vi "GUI.Stream.Disable.vi"(8 "error in (no error)":errorcluster, 11 "State Variables in":T1) -> (0 "error out":errorcluster)   [LabVIEW 2025, in "XNET Bus Monitor Client.lvlib"]
uses:
  XNET Bus Monitor Client.lvlib
  <vilib>/Utility/miscctls.llb/LVRowAndColumnUnsignedTypeDef.ctl
  Types/GUI.StateVariables.ctl
  Types/StreamEngine.CmdQueueData.ctl
  Types/StreamEngine.CmdQueueData.Cmd.ctl
  Types/StreamEngine.QueueRefs.ctl
  Types/GUI.Controls.Refs.ctl
  <vilib>/gRPC/LabVIEW gRPC Library/Shared/grpcId.ctl
  <vilib>/gRPC/LabVIEW gRPC Library/grpc-lvsupport-release.lvlib
  xnet_can_bus_monitor_api_client/RPC Messages/ni_xnet_can_bm_api_DirectionFilter.ctl
  xnet_can_bus_monitor_api_client/xnet_can_bus_monitor_api_client.lvlib
  xnet_can_bus_monitor_api_client/RPC Messages/ni_xnet_can_bm_api_FrameFilter.ctl
  Types/gRPC.ConnectionInfo.ctl
  Types/SubProcessEngine.CmdQueueData.ctl
  Types/SubProcessEngine.CmdQueueData.Cmd.ctl
  Types/SubProcessEngine.QueueRefs.ctl
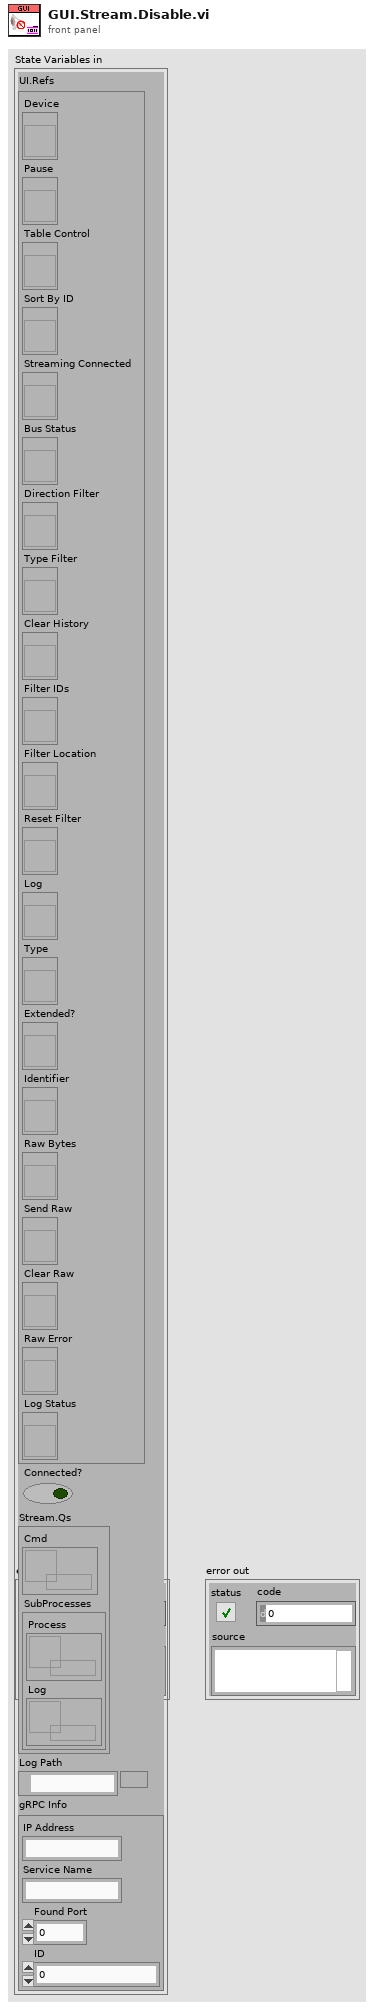
[diagram p1: front panel]
types:
  T1 = typedef "XNET Bus Monitor Client.lvlib/GUI.StateVariables.ctl" = cluster{"UI.Refs":T2, "Connected?":bool, "Stream.Qs":T3, "Log Path":path, "gRPC Info":T5}
  T2 = typedef "XNET Bus Monitor Client.lvlib/GUI.Controls.Refs.ctl" = cluster{"Device":refnum<vi>, "Pause":refnum<vi>, "Table Control":refnum<vi>, "Sort By ID":refnum<vi>, "Streaming Connected":refnum<vi>, "Bus Status":refnum<vi>, "Direction Filter":refnum<vi>, "Type Filter":refnum<vi>, "Clear History":refnum<vi>, "Filter IDs":refnum<vi>, "Filter Location":refnum<vi>, "Reset Filter":refnum<vi>, "Log":refnum<vi>, "Type":refnum<vi>, "Extended?":refnum<vi>, "Identifier":refnum<vi>, "Raw Bytes":refnum<vi>, "Send Raw":refnum<vi>, "Clear Raw":refnum<vi>, "Raw Error":refnum<vi>, "Log Status":refnum<vi>}
  T3 = typedef "XNET Bus Monitor Client.lvlib/StreamEngine.QueueRefs.ctl" = cluster{"Cmd":refnum<queue>, "SubProcesses":T4}
  T4 = typedef "XNET Bus Monitor Client.lvlib/SubProcessEngine.QueueRefs.ctl" = cluster{"Process":refnum<queue>, "Log":refnum<queue>}
  T5 = typedef "XNET Bus Monitor Client.lvlib/gRPC.ConnectionInfo.ctl" = cluster{"IP Address":string, "Service Name":string, "Found Port":u64, "ID":T6}
  T6 = typedef "grpc-lvsupport-release.lvlib/grpcId.ctl" = u64
  T7 = enum16{"CAN Data", "CAN Remote", "CAN Bus Error", "CAN 2.0 Data", "CAN FD Data", "CAN FD+BRS Data", "J1939 Data", "Delay", "Log Trigger", "Start Trigger"}
  T8 = typedef "LVRowAndColumnUnsignedTypeDef.ctl" = cluster{"Row":u32, "Column":u32}
  T9 = enum8{"Enabled", "Disabled", "Disabled and Grayed Out"}
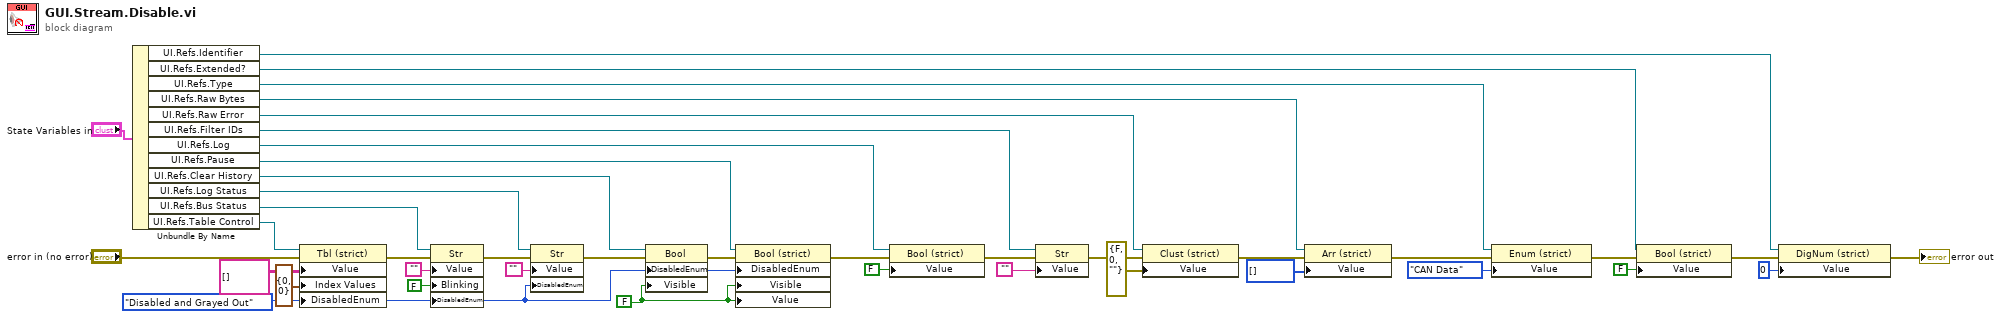
[diagram p0: block diagram]
diagram:
  w30 = FALSE ("Value")
  w3 = T9."Disabled and Grayed Out" ("Disabled")
  n1 = Unbundle By Name("State Variables in") -> ("UI.Refs.Identifier"=w14:refnum<vi>, "UI.Refs.Extended?"=w16:refnum<vi>, "UI.Refs.Type"=w18:refnum<vi>, "UI.Refs.Raw Bytes"=w21:refnum<vi>, "UI.Refs.Raw Error"=w22:refnum<vi>, "UI.Refs.Filter IDs"=w24:refnum<vi>, "UI.Refs.Log"=w28:refnum<vi>, "UI.Refs.Pause"=w31:refnum<vi>, "UI.Refs.Clear History"=w33:refnum<vi>, "UI.Refs.Log Status"=w4:refnum<vi>, "UI.Refs.Bus Status"=w37:refnum<vi>, "UI.Refs.Table Control"=w39:refnum<vi>)
  n2 = property class="Tbl (strict)"(reference=w39, error in="error in (no error)", "Value"=string[][] [], "Index Values"=T8 {"Row"=0, "Column"=0}, "DisabledEnum"=w3) -> (error out=w5:errorcluster)  [unwired: 1 out]
  n3 = property class="Str"(reference=w37, error in=w5, "Value"="", "Blinking"=FALSE, "DisabledEnum"=w3) -> (error out=w2:errorcluster)  [unwired: 1 out]
  n4 = property class="Str"(reference=w4, error in=w2, "Value"="", "DisabledEnum"=w3) -> (error out=w1:errorcluster)  [unwired: 1 out]
  n5 = property class="Bool"(reference=w33, error in=w1, "DisabledEnum"=w3, "Visible"=w30) -> (error out=w32:errorcluster)  [unwired: 1 out]
  n6 = property class="Bool (strict)"(reference=w31, error in=w32, "DisabledEnum"=w3, "Visible"=w30, "Value"=w30) -> (error out=w26:errorcluster)  [unwired: 1 out]
  n7 = property class="Bool (strict)"(reference=w28, error in=w26, "Value"=FALSE ("Visible")) -> (error out=w25:errorcluster)  [unwired: 1 out]
  n8 = property class="Str"(reference=w24, error in=w25, "Value"="") -> (error out=w20:errorcluster)  [unwired: 1 out]
  n9 = property class="Clust (strict)"(reference=w22, error in=w20, "Value"=errorcluster {"status"=FALSE, "code"=0, "source"=""}) -> (error out=w19:errorcluster)  [unwired: 1 out]
  n10 = property class="Arr (strict)"(reference=w21, error in=w19, "Value"=u8[] []) -> (error out=w17:errorcluster)  [unwired: 1 out]
  n11 = property class="Enum (strict)"(reference=w18, error in=w17, "Value"=T7."CAN Data") -> (error out=w15:errorcluster)  [unwired: 1 out]
  n12 = property class="Bool (strict)"(reference=w16, error in=w15, "Value"=FALSE) -> (error out=w13:errorcluster)  [unwired: 1 out]
  n13 = property class="DigNum (strict)"(reference=w14, error in=w13, "Value"=u32 0) -> (error out=→"error out":errorcluster)  [unwired: 1 out]
